vi "Main.vi"() -> ()   [LabVIEW 2017]
uses:
  1. CTL/DAQ_AO.ctl
  1. CTL/Controller.ctl
  <vilib>/DAQmx/read.llb/DAQmx Read (Analog 1D DBL 1Chan NSamp).vi
  <vilib>/Analysis/_algsub.llb/Real Vector Norm.vi
  <vilib>/DAQmx/write.llb/DAQmx Write (Digital Bool 1Line 1Point).vi
  <vilib>/DAQmx/write.llb/DAQmx Write (Analog 1D DBL 1Chan NSamp).vi
  <vilib>/DAQmx/write.llb/DAQmx Write (Analog 2D DBL NChan NSamp).vi
  <vilib>/Analysis/2dsp.llb/Decimate (single shot, DBL).vi
  <vilib>/DAQmx/create/channels.llb/DAQmx Create Channel (AO-Voltage-Basic).vi
  <vilib>/DAQmx/create/channels.llb/DAQmx Create Channel (AI-Voltage-Basic).vi
  <vilib>/DAQmx/configure/timing.llb/DAQmx Timing (Sample Clock).vi
  <vilib>/DAQmx/create/channels.llb/DAQmx Create Channel (DO-Digital Output).vi
  <vilib>/DAQmx/configure/trigger.llb/DAQmx Start Trigger (Analog Edge).vi
  <vilib>/DAQmx/miscellaneous.llb/DAQmx Fill In Error Info.vi
  <vilib>/Analysis/2dsp.llb/1D Cross Correlation (DBL).vi
  <vilib>/Analysis/NI_AALPro.lvlib
  <vilib>/Analysis/NI_AALBase.lvlib
panel:
  out "수신 신호 파형(PPM)":waveform(dbl)(graph)
  out "수신 신호 파형":waveform(dbl)(graph)
  out "최대값 3":dbl
  out "신호처리 파형(PPM)":waveform(dbl)(graph)
  out "최대값 2":dbl
  in  "Tab Control":T1(tab)
  in  "일시 정지 버튼":bool
  out "송신 신호생성 파형":waveform(dbl)[](graph)
  out "신호처리파형":waveform(dbl)(graph)
  out "최대값":dbl
  out "이전 최대값":dbl
  out "최대값 차이":dbl
  in  "정지 버튼":bool
  in  "수동시작 버튼":bool
  in  "자동시작 버튼":bool
  in  "Chip_rate_Threshold":u32(knob)=10 scale=0.0..20.0
  in  "Threshold":u32(knob)=10 scale=0.0..20.0
  in  "수신시간":dbl=0.5
  in  "Rc":dbl=5500.0 min=4000.0 step=100.0
  in  "Mask 데이터 참조 경로":string="C:\\Users\\FishingNetID\\Desktop\\TRX_CONTROLLER_SIMULATRO_1.4\\3. TDMS\\Coef8.tdms"
  in  "TX_Period":dbl=3.0
  in  "Mask 길이":enum16{"8 Order", "12 Order"}(ring)
  in  "주소":string="192.168.0.147"
  in  "원격 포트 또는 서비스 이름":u16=10000
  out "원소":T2
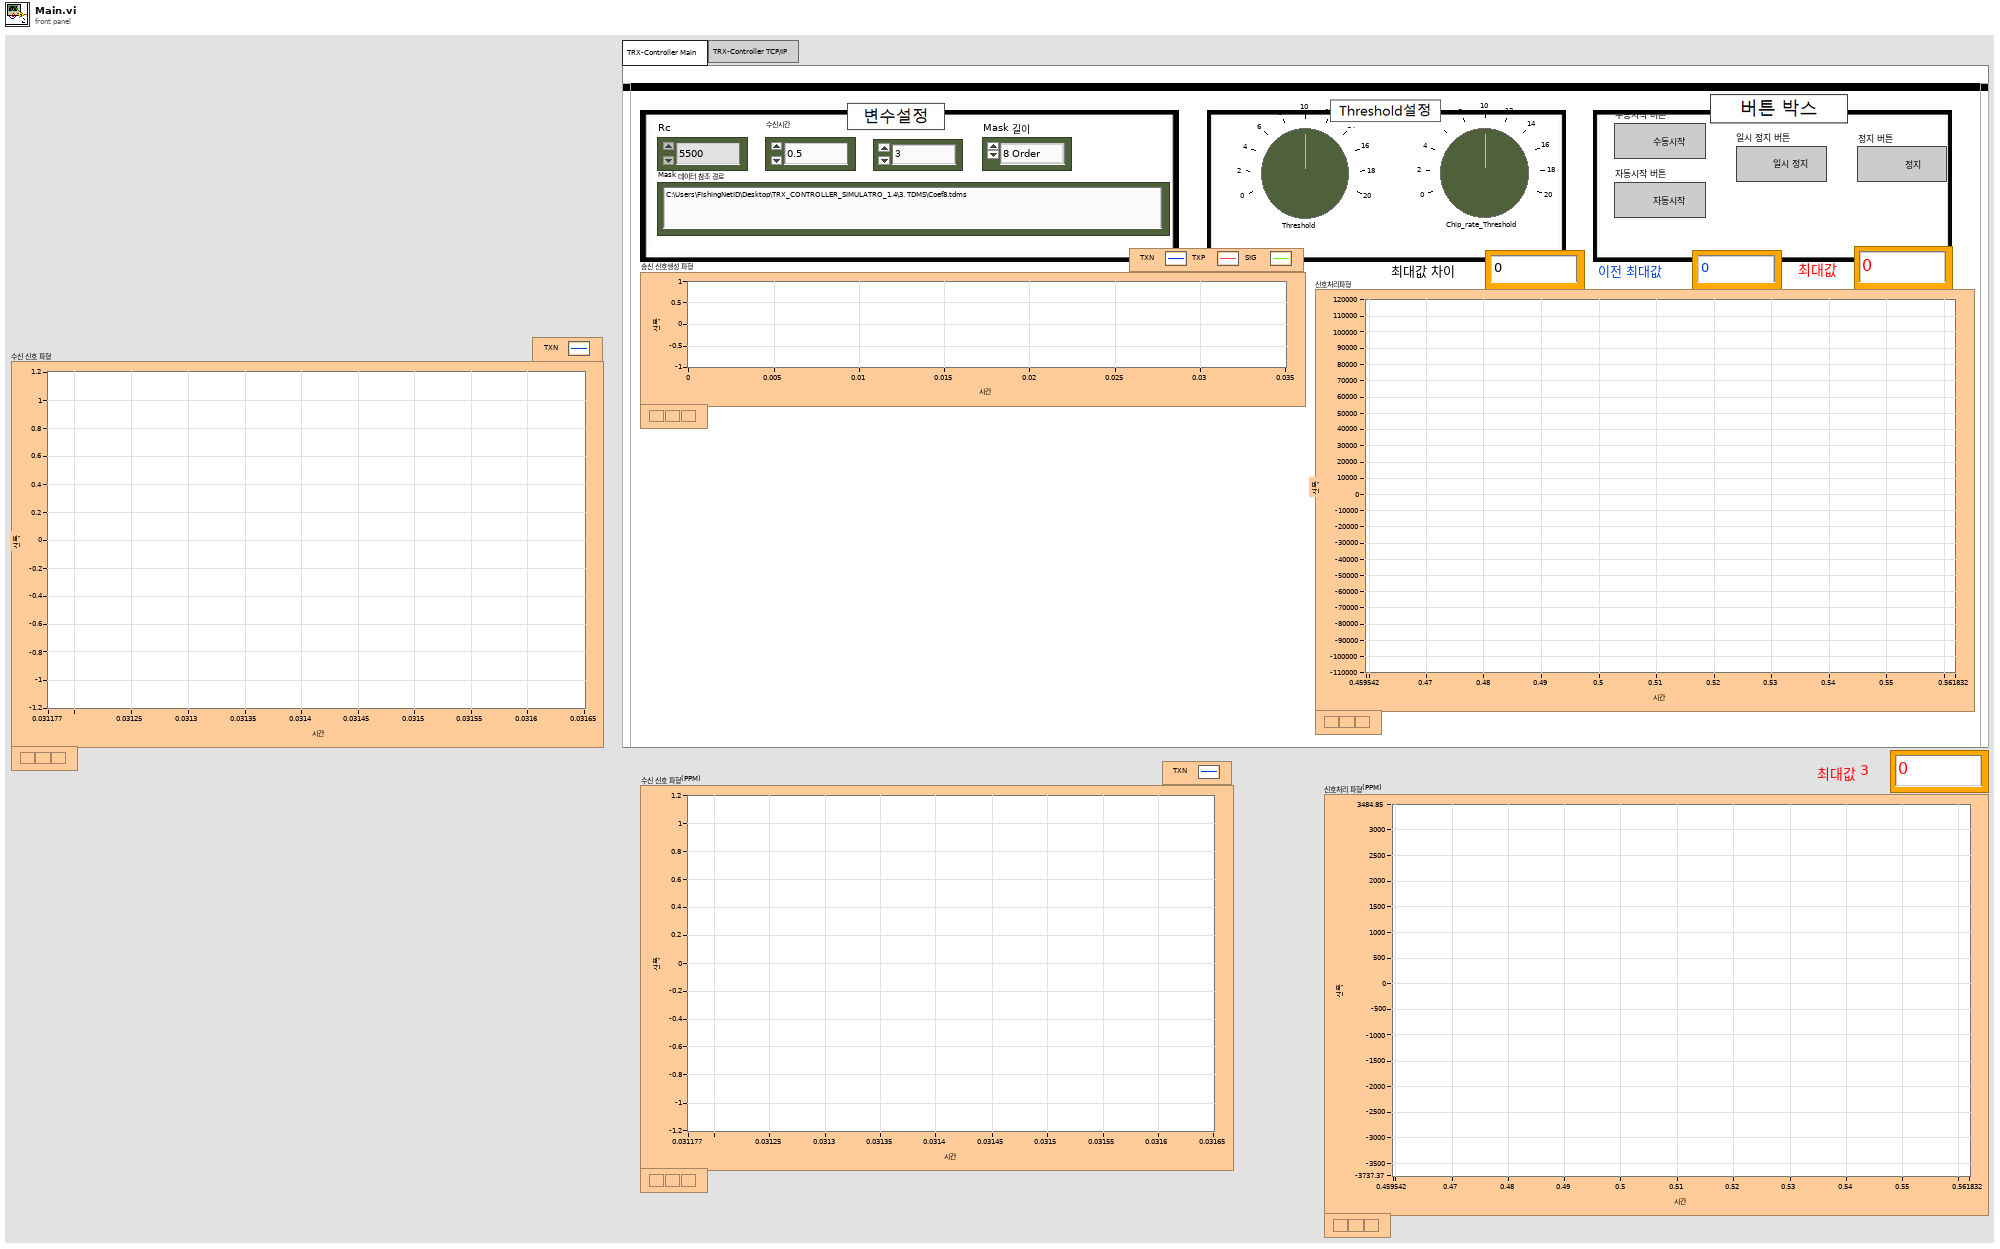
[diagram p1: front panel]
types:
  T1 = enum32{"TRX-Controller Main", "TRX-Controller TCP/IP"}
  T2 = typedef "DAQ_AO.ctl" = enum16{"통신 초기화", "통신 시작", "통신 정지"}
  T3 = cluster{"연결 ID":refnum<k5>, "TCP 에러":errorcluster}
  T4 = cluster{"송신신호 생성":waveform(dbl)[], "TXP 신호":dbl[], "TXN 신호":dbl[], "Fs":dbl, "AI 참조":refnum<k21>, "AO 참조":refnum<k21>, "수신시간":dbl, "Rc":dbl, "이전 최대값":dbl, "수신 신호처리 파형":waveform(dbl), "수신 파형":waveform(dbl), "최대값":dbl, "최대값 차이":dbl, "DO 참조":refnum<k21>, "TXEN 신호":bool[]}
  T5 = typedef "Controller.ctl" = enum16{"초기화", "수동시작", "신호처리", "정지", "값 변경", "일시정지", "자동시작"}
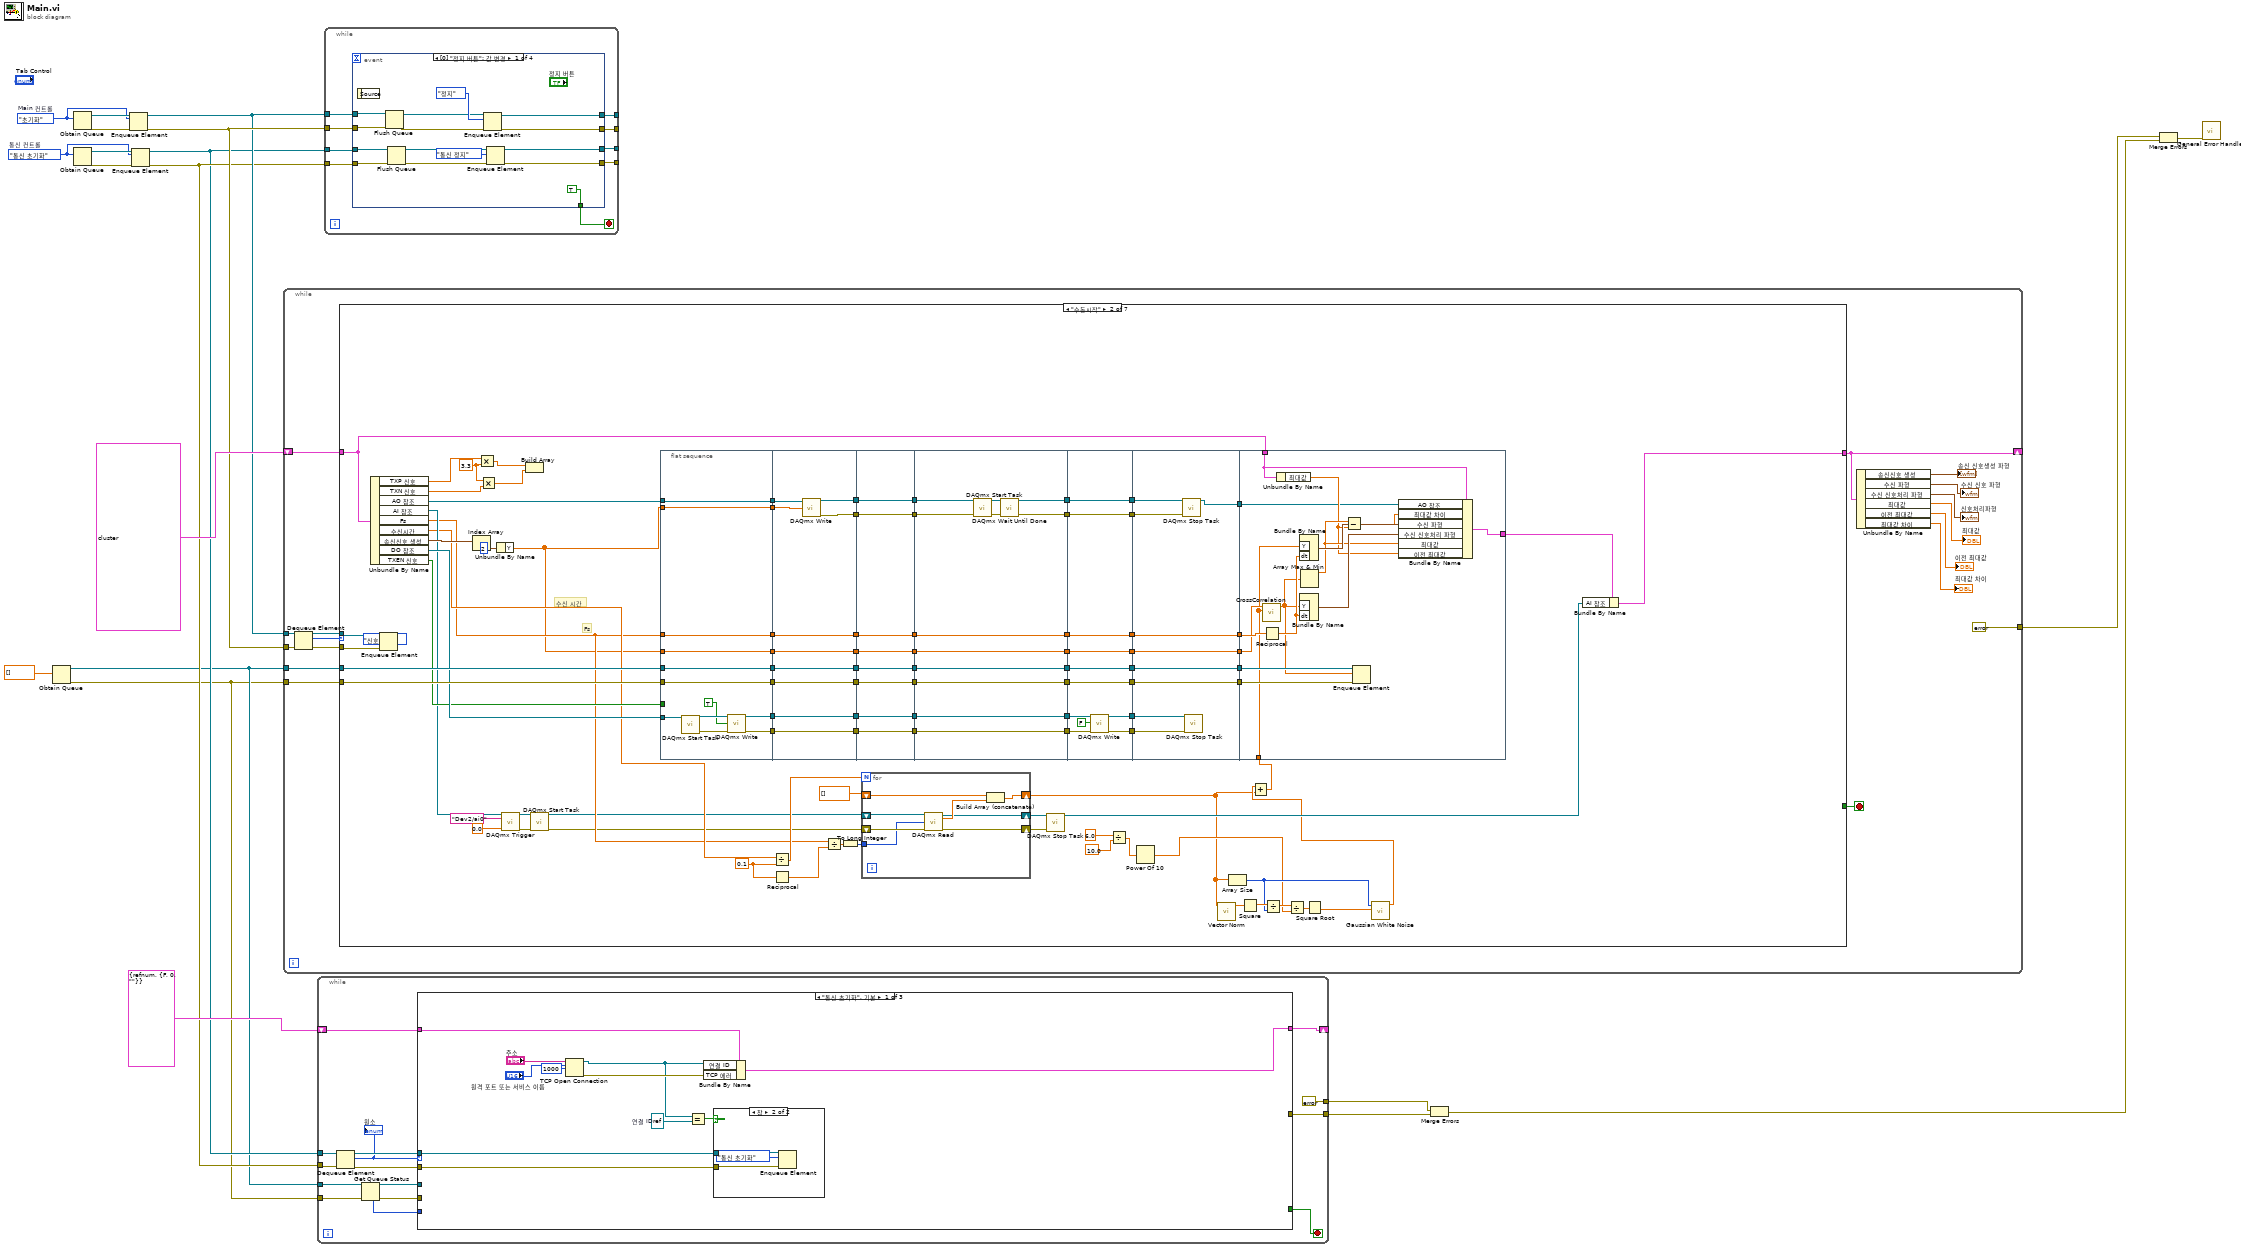
[diagram p0: block diagram]
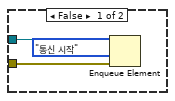
[diagram p2: hidden frame]
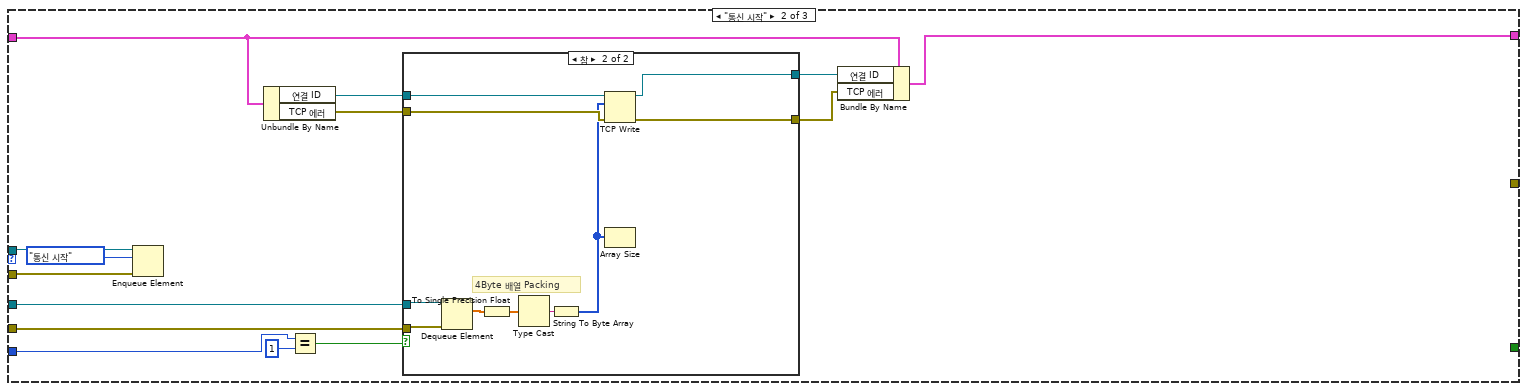
[diagram p3: hidden frame]
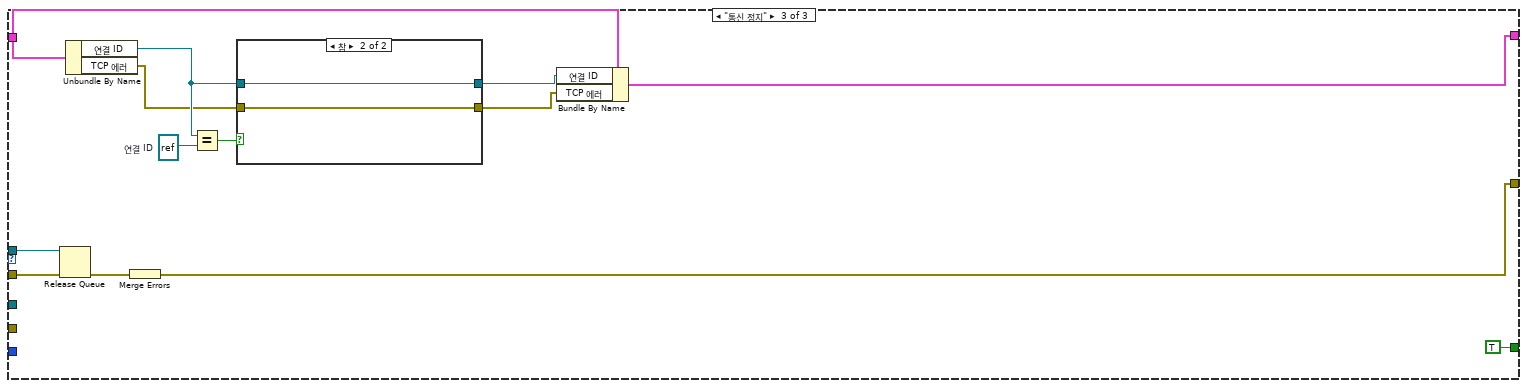
[diagram p5: hidden frame]
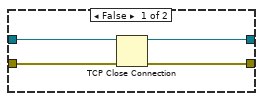
[diagram p6: hidden frame]
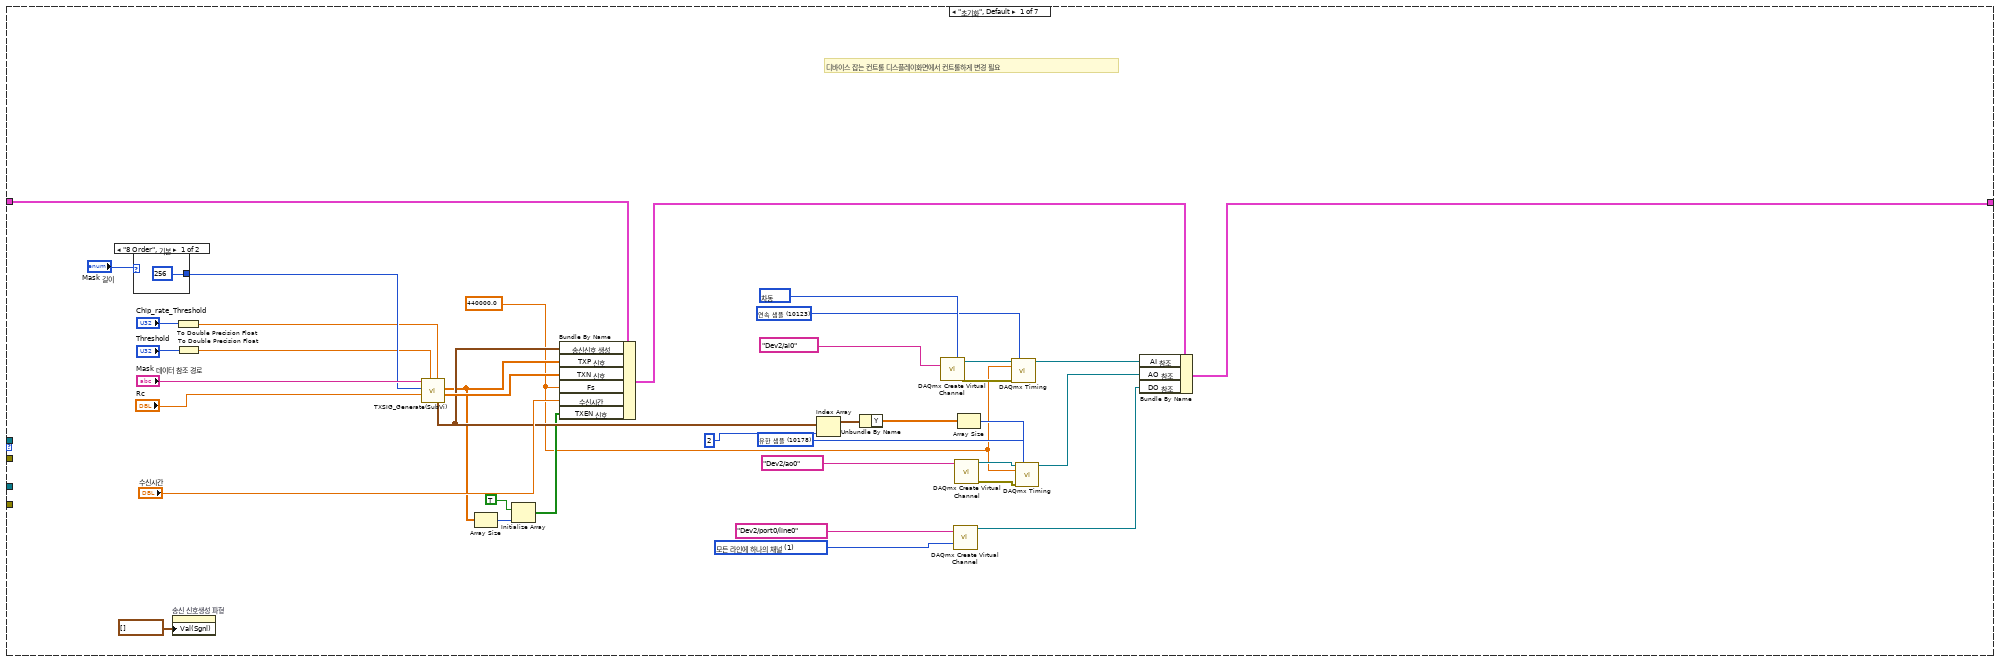
[diagram p7: hidden frame]
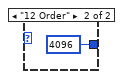
[diagram p8: hidden frame]
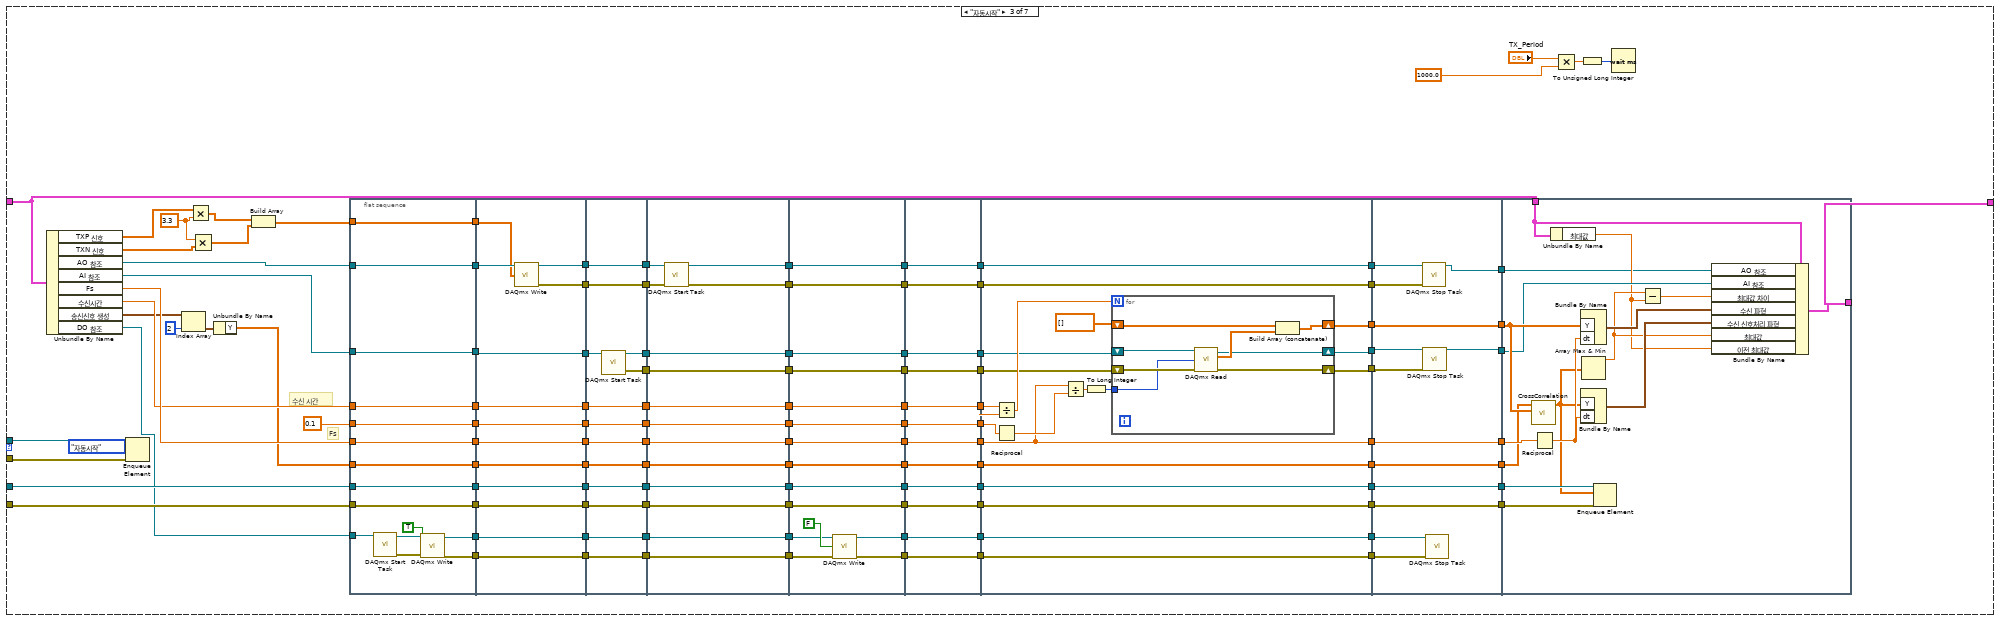
[diagram p9: hidden frame]
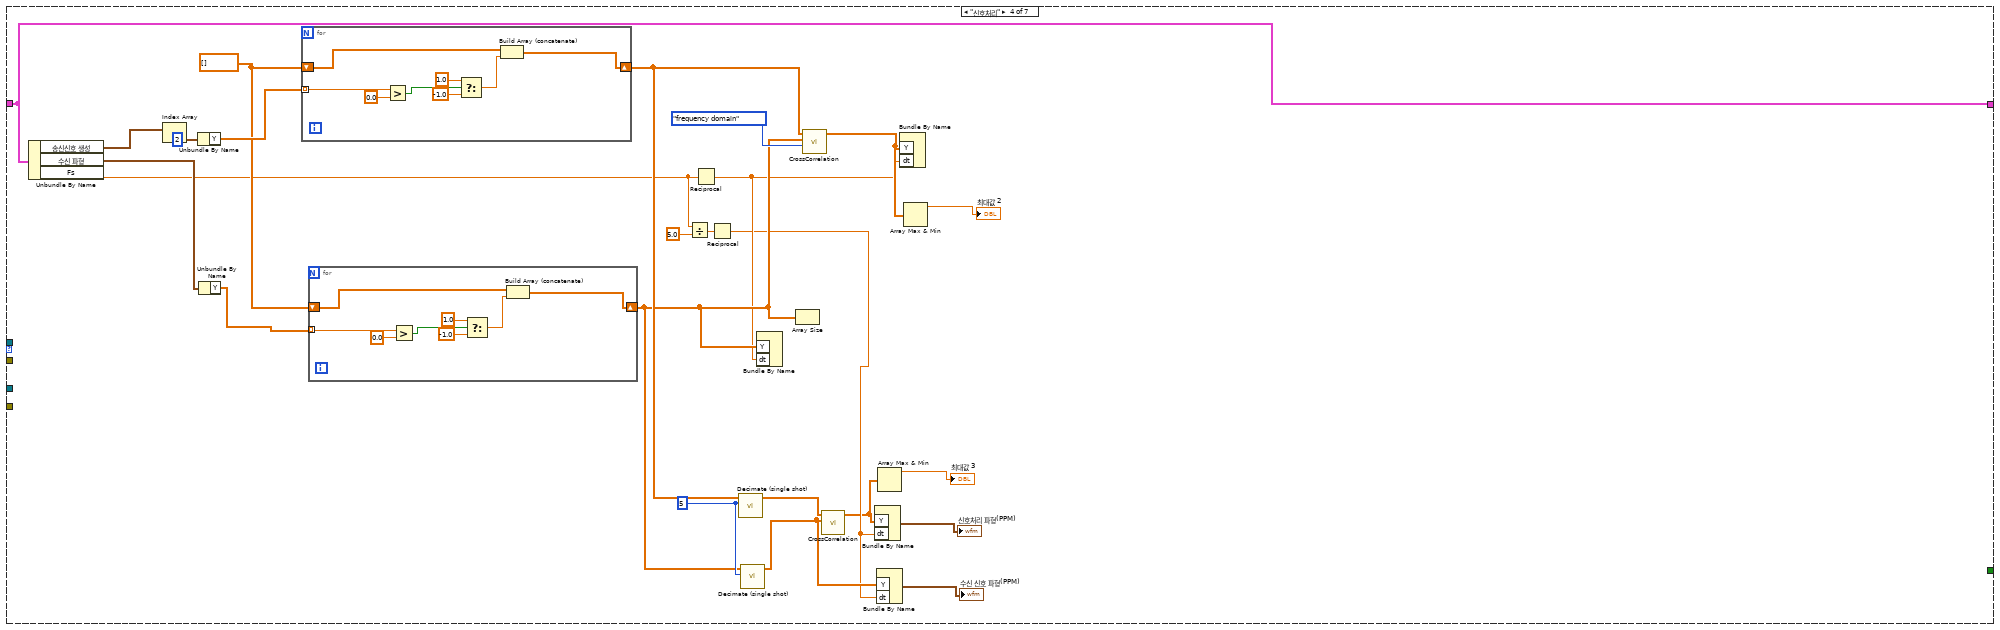
[diagram p10: hidden frame]
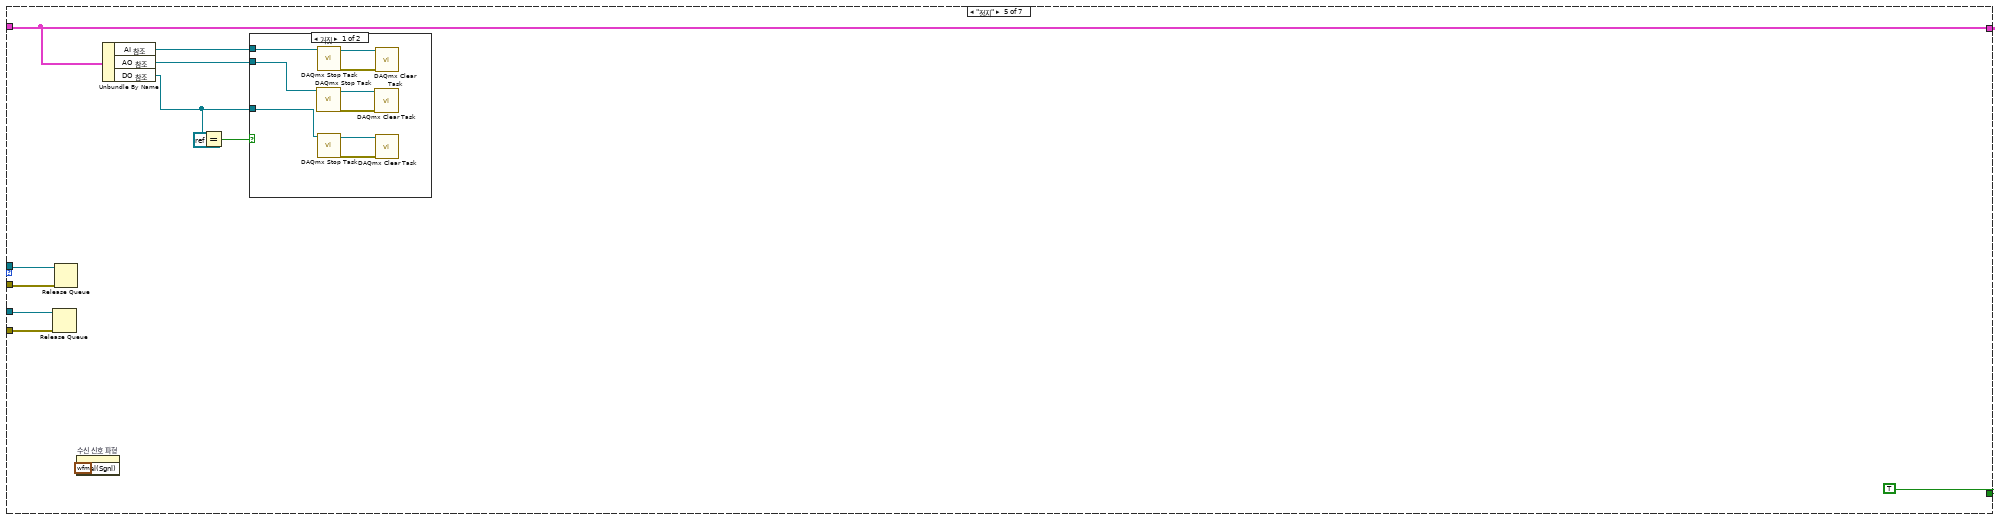
[diagram p11: hidden frame]
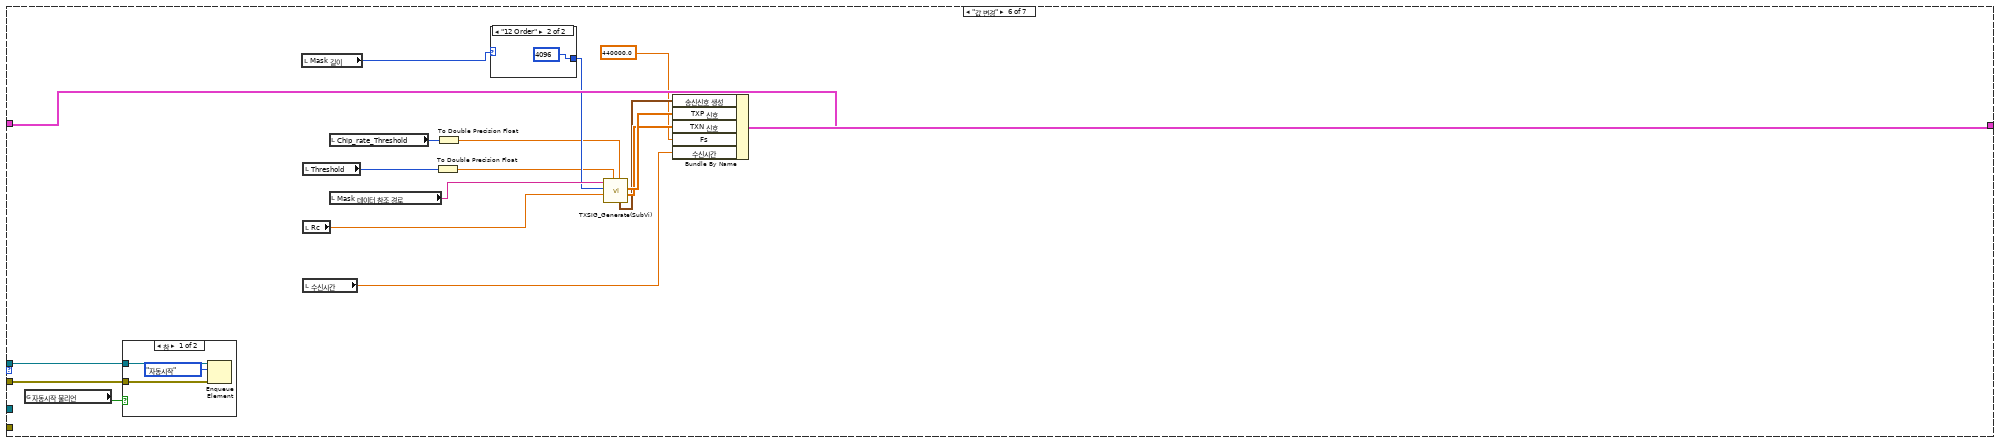
[diagram p13: hidden frame]
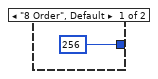
[diagram p14: hidden frame]
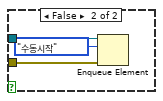
[diagram p15: hidden frame]
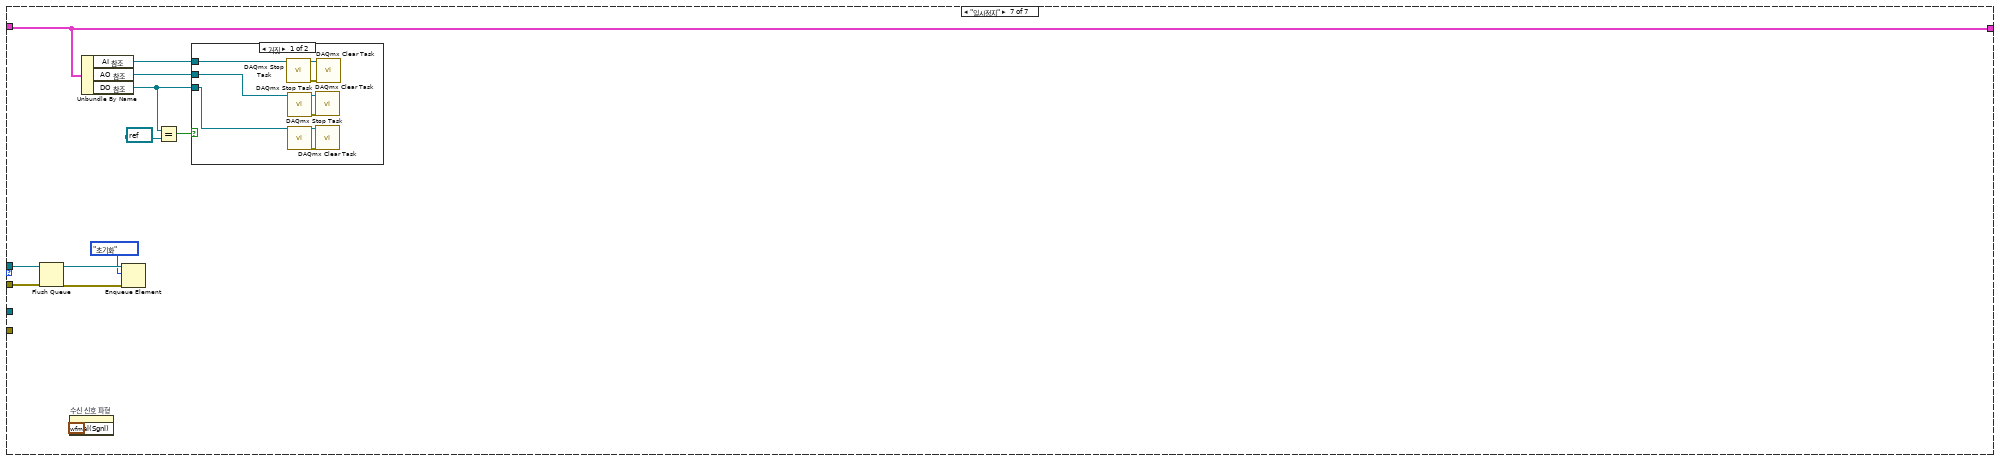
[diagram p16: hidden frame]
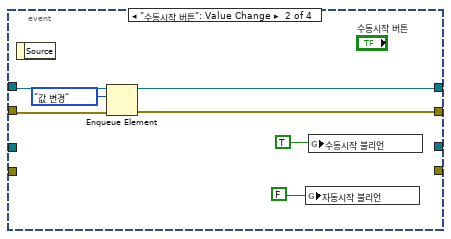
[diagram p18: hidden frame]
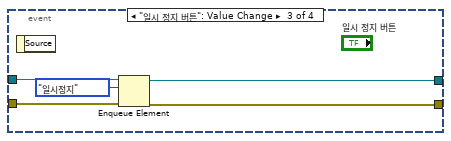
[diagram p19: hidden frame]
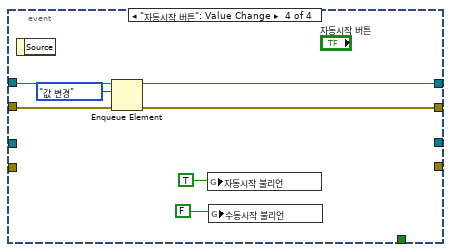
[diagram p20: hidden frame]
diagram:
  w8 = DAQ_AO."통신 초기화"  # 통신 컨트롤
  w15 = Controller."초기화"  # Main 컨트롤
  n1 = Obtain Queue(element data type=dbl[] []) -> (queue out=w2:refnum<queue>, error out=w1:errorcluster)  [unwired: 4 in, 1 out]
  n2 = Obtain Queue(element data type=w8) -> (queue out=w12:refnum<queue>, error out=w11:errorcluster)  [unwired: 4 in, 1 out]
  n3 = Obtain Queue(element data type=w15) -> (queue out=w19:refnum<queue>, error out=w18:errorcluster)  [unwired: 4 in, 1 out]
  n4 = Enqueue Element(queue=w19, element=w15, error in (no error)=w18) -> (queue out=w16:refnum<queue>, error out=w17:errorcluster)  [unwired: 1 in, 1 out]
  n5 = Enqueue Element(queue=w12, element=w8, error in (no error)=w11) -> (queue out=w9:refnum<queue>, error out=w10:errorcluster)  [unwired: 1 in, 1 out]
  n6 = while {
    tunnel: w16 -> [w37]
    tunnel: w17 -> [w36]
    tunnel: [errorcluster {"status"=FALSE, "code"=0, "source"=""} ("에러 상수")] -> w3
    shift-right: [w30] -> _
    shift-left: T4 {"송신신호 생성"=[], "TXP 신호"=[], "TXN 신호"=[], "Fs"=0.0, "AI 참조"="", "AO 참조"="", "수신시간"=0.0, "Rc"=0.0, "이전 최대값"=0.0, "수신 신호처리 파형"={"t0"=timestamp(0 s since 1904-01-01), "dt"=1.0, "Y"=[]}, "수신 파형"={"t0"=timestamp(0 s since 1904-01-01), "dt"=1.0, "Y"=[]}, "최대값"=0.0, "최대값 차이"=0.0, "DO 참조"="", "TXEN 신호"=[]} -> [w31]
    tunnel: w2 -> [w23]
    tunnel: w1 -> [w22]
    stop <- w34 stop-if-true
    n7 = Dequeue Element(queue=w37, error in (no error)=w36) -> (queue out=w33:refnum<queue>, element=w21:T5, error out=w32:errorcluster)  [unwired: 1 in, 1 out]
    n8 = case shown="\"수동시작\"" w21 {
      tunnel: [_ _ _ _ TRUE _ _] -> w34
      tunnel: w31 -> [w72 w172 w366 w531 w564 w584 w606]
      tunnel: [w73 w93 w345 w531 w564 w588 w606] -> w30
      tunnel: w33 -> [_ w135 w344 _ w555 w586 w612]
      tunnel: w32 -> [_ w134 w343 _ w554 w585 w611]
      tunnel: w23 -> [_ w162 w341 _ w557 _ _]
      tunnel: w22 -> [_ w160 w340 _ w556 _ _]
      frame "초기화", Default {
        w45 = 1 items=["각 라인에 하나의 채널", "모든 라인에 하나의 채널"] ("line grouping")
        w38 = 440000.0 ("Fs")
        w70 = 10106 items=["기본"=-1, "RSE"=10083, "NRSE"=10078, "차동"=10106, "유사 차동"=12529] ("input terminal configuration")
        w64 = 10178 items=["유한 샘플"=10178, "연속 샘플"=10123, "하드웨어 타이밍에 의한 단일 포인트"=12522] ("sample mode")
        w67 = 10123 items=["유한 샘플"=10178, "연속 샘플"=10123, "하드웨어 타이밍에 의한 단일 포인트"=12522] ("sample mode")
        # "디바이스 잡는 컨트롤 디스플레이화면에서 컨트롤하게 변경 필요"
        n9 = case shown="\"8 Order\", 기본" "Mask 길이" {
          tunnel: [256 4096] -> w55
          frame "8 Order", Default {
          }
          frame "12 Order" {
          }
        }
        n10 = property on="송신 신호생성 파형" class="WFGraph (엄격한)"("Val(Sgnl)"=waveform(dbl)[] []) -> ()  [unwired: 2 in, 2 out]
        n11 = To Double Precision Float(number="Chip_rate_Threshold") -> (double precision float=w53:dbl)
        n12 = To Double Precision Float(number="Threshold") -> (double precision float=w51:dbl)
        n13 = call "TXSIG_Generate(SubVi).vi"("Chip_rate_Threshold"=w53, "ThresHold"=w51, "Rc"="Rc", "길이"=w55, "이름 또는 상대 경로"="Mask 데이터 참조 경로") -> ("TXN"=w59:dbl[], "TXP"=w43:dbl[], "TXSIG"=w47:waveform(dbl)[])  [unwired: 4 in]
        n14 = Array Size(array=w43) -> (size(s)=w42:i32)
        n15 = Initialize Array(TRUE, w42) -> (w40:bool[])
        n16 = Bundle By Name(cluster=w72, "송신신호 생성"=w47, "TXP 신호"=w43, "TXN 신호"=w59, "Fs"=w38, "수신시간"="수신시간", "TXEN 신호"=w40) -> (w71:T4)
        n17 = Index Array(array=w47, index=2 ("인덱스")) -> (element=w49:waveform(dbl))
        n18 = Unbundle By Name(w49) -> ("Y"=w48:dbl[])
        n19 = call-poly <vilib>:"DAQmx Create Virtual Channel.vi"("input terminal configuration"=w70, "physical channels"=tag "Dev2/ai0") -> ("task out"=w69:refnum<k21>, "error out"=w68:errorcluster)  [unwired: 12 in]
        n20 = call-poly <vilib>:"DAQmx Create Virtual Channel.vi"("lines"=tag "Dev2/port0/line0", "line grouping"=w45) -> ("task out"=w44:refnum<k21>)  [unwired: 12 in, 1 out]
        n21 = call-poly <vilib>:"DAQmx Create Virtual Channel.vi"("physical channels"=tag "Dev2/ao0") -> ("task out"=w65:refnum<k21>, "error out"=w62:errorcluster)  [unwired: 13 in]
        n22 = Array Size(array=w48) -> (size(s)=w61:i32)
        n23 = call-poly <vilib>:"DAQmx Timing.vi"("task/channels in"=w69, "sample mode"=w67, "rate"=w38, "error in"=w68) -> ("task out"=w66:refnum<k21>)  [unwired: 10 in, 1 out]
        n24 = call-poly <vilib>:"DAQmx Timing.vi"("task/channels in"=w65, "sample mode"=w64, "samples per channel"=w61, "rate"=w38, "error in"=w62) -> ("task out"=w63:refnum<k21>)  [unwired: 9 in, 1 out]
        n25 = Bundle By Name(cluster=w71, "AI 참조"=w66, "AO 참조"=w63, "DO 참조"=w44) -> (w73:T4)
      }
      frame "수동시작" {
        w105 = 0.1 ("y")
        w167 = 3.3
        # "Fs"
        # "수신 시간"
        n26 = Unbundle By Name(w172) -> ("TXP 신호"=w169:dbl[], "TXN 신호"=w168:dbl[], "AO 참조"=w173:refnum<k21>, "AI 참조"=w113:refnum<k21>, "Fs"=w104:dbl, "수신시간"=w106:dbl, "송신신호 생성"=w165:waveform(dbl)[], "DO 참조"=w158:refnum<k21>, "TXEN 신호"=w142:bool[])
        n27 = Enqueue Element(queue=w135, element=Controller."신호처리" ("원소"), error in (no error)=w134) -> ()  [unwired: 1 in, 3 out]
        n28 = Index Array(array=w165, index=2 ("인덱스")) -> (element=w171:waveform(dbl))
        n29 = Multiply(x=w169, y=w167) -> (x*y=w143:dbl[])
        n30 = Multiply(x=w167, y=w168) -> (x*y=w166:dbl[])
        n31 = Unbundle By Name(w171) -> ("Y"=w91:dbl[])
        n32 = call-poly <vilib>:"DAQmx Trigger.vi"("task/channels in"=w113, "source"="Dev2/ai0", "level"=0.0) -> ("task out"=w115:refnum<k21>, "error out"=w114:errorcluster)  [unwired: 11 in]
        n33 = Build Array(w143, w166) -> ()  [unwired: 1 out]
        n34 = call <vilib>:"DAQmx Start Task.vi"("task/channels in"=w115, "error in"=w114) -> ("task out"=w103:refnum<k21>, "error out"=w102:errorcluster)  [unwired: 12 in]
        n35 = flat-sequence {
          tunnel: w158 -> [w187]
          tunnel: w160 -> [w188]
          tunnel: w162 -> [w189]
          tunnel: w91 -> [w190]
          tunnel: w91 -> [w191]
          tunnel: w104 -> [w192]
          tunnel: w173 -> [w193]
          tunnel: [w193] -> w157
          tunnel: [w192] -> w156
          tunnel: [w191] -> w155
          tunnel: [w190] -> w154
          tunnel: [w189] -> w153
          tunnel: [w188] -> w152
          tunnel: [w184] -> w147
          tunnel: [w183] -> w146
          tunnel: w142 -> [_]
          tunnel: [w202] -> w118
          tunnel: [w201] -> w120
          tunnel: [w200] -> w122
          tunnel: [w198] -> w124
          tunnel: [w197] -> w126
          tunnel: [w196] -> w128
          tunnel: w157 -> [w203]
          tunnel: w156 -> [w200]
          tunnel: w155 -> [w199]
          tunnel: w154 -> [w198]
          tunnel: w153 -> [w197]
          tunnel: w152 -> [w196]
          tunnel: [w195] -> w130
          tunnel: w147 -> [w195]
          tunnel: w146 -> [w194]
          tunnel: [w194] -> w132
          tunnel: w132 -> [w211]
          tunnel: [w211] -> w131
          tunnel: w130 -> [w210]
          tunnel: [w210] -> w129
          tunnel: w128 -> [w209]
          tunnel: [w209] -> w127
          tunnel: w126 -> [w208]
          tunnel: [w208] -> w125
          tunnel: w124 -> [w207]
          tunnel: [w207] -> w123
          tunnel: w122 -> [w206]
          tunnel: [w206] -> w121
          tunnel: w120 -> [w205]
          tunnel: [w205] -> w119
          tunnel: w118 -> [w204]
          tunnel: [w204] -> w117
          tunnel: [w223] -> w141
          tunnel: [w222] -> w140
          tunnel: [w221] -> w139
          tunnel: [w220] -> w138
          tunnel: [w219] -> w137
          tunnel: [w218] -> w136
          tunnel: w131 -> [w218]
          tunnel: w129 -> [w219]
          tunnel: w127 -> [w220]
          tunnel: w125 -> [w221]
          tunnel: w123 -> [w222]
          tunnel: w121 -> [w223]
          tunnel: w119 -> [w217]
          tunnel: w117 -> [w216]
          tunnel: [w213] -> w98
          tunnel: [w212] -> w97
          tunnel: w141 -> [w234]
          tunnel: [w234] -> w151
          tunnel: w140 -> [w233]
          tunnel: [w233] -> w150
          tunnel: w139 -> [w232]
          tunnel: [w232] -> w149
          tunnel: w138 -> [w231]
          tunnel: [w231] -> w148
          tunnel: w137 -> [w230]
          tunnel: w136 -> [w229]
          tunnel: [w228] -> w145
          tunnel: [w227] -> w144
          tunnel: [w225] -> w99
          tunnel: w98 -> [w225]
          tunnel: w97 -> [w224]
          tunnel: [w224] -> w96
          tunnel: [w243] -> w164
          tunnel: [w242] -> w163
          tunnel: [w241] -> w161
          tunnel: [w240] -> w159
          tunnel: [w237] -> w116
          tunnel: w151 -> [w243]
          tunnel: w150 -> [w242]
          tunnel: w149 -> [w241]
          tunnel: w148 -> [w240]
          tunnel: w145 -> [w239]
          tunnel: w144 -> [w238]
          tunnel: w99 -> [w236]
          tunnel: w96 -> [w235]
          tunnel: w172 -> [w255]
          tunnel: w164 -> [w257]
          tunnel: w163 -> [w256]
          tunnel: [w252] -> w95
          tunnel: w161 -> [w248]
          tunnel: w159 -> [w247]
          tunnel: w116 -> [w245]
          tunnel: w79 -> [w244]
          frame #0 {
            n36 = call <vilib>:"DAQmx Start Task.vi"("task/channels in"=w187) -> ("task out"=w186:refnum<k21>, "error out"=w185:errorcluster)  [unwired: 13 in]
            n37 = call-poly <vilib>:"DAQmx Write.vi"("task/channels in"=w186, "data"=TRUE, "error in"=w185) -> ("task out"=w184:refnum<k21>, "error out"=w183:errorcluster)  [unwired: 10 in, 1 out]
          }
          frame #1 {
            n38 = call-poly <vilib>:"DAQmx Write.vi"("task/channels in"=w203, "data"=w199) -> ("task out"=w202:refnum<k21>, "error out"=w201:errorcluster)  [unwired: 11 in, 1 out]
          }
          frame #2 {
          }
          frame #3 {
            n39 = call <vilib>:"DAQmx Start Task.vi"("task/channels in"=w216, "error in"=w217) -> ("task out"=w215:refnum<k21>, "error out"=w214:errorcluster)  [unwired: 12 in]
            n40 = call <vilib>:"DAQmx Wait Until Done.vi"("task/channels in"=w215, "error in"=w214) -> ("task out"=w213:refnum<k21>, "error out"=w212:errorcluster)  [unwired: 12 in]
          }
          frame #4 {
            n41 = call-poly <vilib>:"DAQmx Write.vi"("task/channels in"=w230, "data"=FALSE, "error in"=w229) -> ("task out"=w228:refnum<k21>, "error out"=w227:errorcluster)  [unwired: 10 in, 1 out]
          }
          frame #5 {
            n42 = call <vilib>:"DAQmx Stop Task.vi"("task/channels in"=w236, "error in"=w235) -> ("task out"=w237:refnum<k21>)  [unwired: 12 in, 1 out]
            n43 = call <vilib>:"DAQmx Stop Task.vi"("task/channels in"=w239, "error in"=w238) -> ()  [unwired: 12 in, 2 out]
          }
          frame #6 {
            n44 = call-poly <vilib>:"CrossCorrelation.vi"("Y"=w244, "X"=w256) -> ("Rxy"=w246:dbl[])  [unwired: 8 in, 1 out]
            n45 = Reciprocal(x=w257) -> (1/x=w258:dbl)
            n46 = Unbundle By Name(w255) -> ("최대값"=w249:dbl)
            n47 = Bundle By Name("Y"=w244, "dt"=w258) -> (w254:waveform(dbl))  [unwired: 1 in]
            n48 = Bundle By Name("Y"=w246, "dt"=w258) -> (w253:waveform(dbl))  [unwired: 1 in]
            n49 = Array Max & Min(array=w246) -> (max value=w250:dbl)  [unwired: 3 out]
            n50 = Subtract(x=w250, y=w249) -> (x-y=w251:dbl)
            n51 = Enqueue Element(queue=w248, element=w246, error in (no error)=w247) -> ()  [unwired: 1 in, 3 out]
            n52 = Bundle By Name(cluster=w255, "AO 참조"=w245, "최대값 차이"=w251, "수신 파형"=w254, "수신 신호처리 파형"=w253, "최대값"=w250, "이전 최대값"=w249) -> (w252:T4)
          }
        }
        n53 = Divide(x=w106, y=w105) -> (x/y=w108:dbl)
        n54 = Reciprocal(x=w105) -> (1/x=w109:dbl)
        n55 = Divide(x=w104, y=w109) -> (x/y=w111:dbl)
        n56 = To Long Integer(number=w111) -> (32bit integer=w110:i32)
        n57 = for {
          N: w108 -> [_]
          shift-right: [w179] -> w80
          shift-left: dbl[] [] -> [w181]
          shift-right: [w175] -> w101
          shift-left: w103 -> [w178]
          shift-right: [w176] -> w100
          shift-left: w102 -> [w177]
          tunnel: w110 -> [w174]
          n58 = call-poly <vilib>:"DAQmx Read.vi"("task/channels in"=w178, "number of samples per channel"=w174, "error in"=w177) -> ("task out"=w175:refnum<k21>, "data"=w180:dbl[], "error out"=w176:errorcluster)  [unwired: 10 in]
          n59 = Build Array (concatenate)(w181, w180) -> (w179:dbl[])
        }
        n60 = call <vilib>:"DAQmx Stop Task.vi"("task/channels in"=w101, "error in"=w100) -> ("task out"=w94:refnum<k21>)  [unwired: 12 in, 1 out]
        n61 = Divide(x=6.0, y=10.0) -> (x/y=w83:dbl)
        n62 = Power Of 10(x=w83) -> (10^x=w82:dbl)
        n63 = call-poly <vilib>:"Vector Norm.vi"("Input Vector"=w80) -> ("norm"=w89:dbl)  [unwired: 9 in, 1 out]
        n64 = Array Size(array=w80) -> (size(s)=w85:i32)
        n65 = Square(x=w89) -> (x^2=w88:dbl)
        n66 = Divide(x=w88, y=w85) -> (x/y=w87:dbl)
        n67 = Divide(x=w87, y=w82) -> (x/y=w86:dbl)
        n68 = Square Root(x=w86) -> (sqrt(x)=w84:dbl)
        n69 = call <vilib>:"Gaussian White Noise.vi"("standard deviation"=w84, "samples"=w85) -> ("Gaussian noise pattern"=w81:dbl[])  [unwired: 8 in, 1 out]
        n70 = Add(x=w81, y=w80) -> (x+y=w79:dbl[])
        n71 = Bundle By Name(cluster=w95, "AI 참조"=w94) -> (w93:T4)
      }
      frame "자동시작" {
        w358 = 3.3
        # "Fs"
        # "수신 시간"
        n72 = Unbundle By Name(w366) -> ("TXP 신호"=w360:dbl[], "TXN 신호"=w359:dbl[], "AO 참조"=w373:refnum<k21>, "AI 참조"=w354:refnum<k21>, "Fs"=w372:dbl, "수신시간"=w369:dbl, "송신신호 생성"=w355:waveform(dbl)[], "DO 참조"=w319:refnum<k21>)
        n73 = Enqueue Element(queue=w344, element=Controller."자동시작" ("원소"), error in (no error)=w343) -> ()  [unwired: 1 in, 3 out]
        n74 = Index Array(array=w355, index=2 ("인덱스")) -> (element=w362:waveform(dbl))
        n75 = Multiply(x=w360, y=w358) -> (x*y=w357:dbl[])
        n76 = Multiply(x=w358, y=w359) -> (x*y=w356:dbl[])
        n77 = Unbundle By Name(w362) -> ("Y"=w349:dbl[])
        n78 = Build Array(w357, w356) -> (w333:dbl[][])
        n79 = flat-sequence {
          tunnel: w333 -> [w380]
          tunnel: w340 -> [w381]
          tunnel: w341 -> [w382]
          tunnel: w349 -> [w383]
          tunnel: 0.1 ("y") -> [w384]
          tunnel: w369 -> [w385]
          tunnel: w372 -> [w386]
          tunnel: w354 -> [w387]
          tunnel: w373 -> [w388]
          tunnel: [w388] -> w328
          tunnel: [w387] -> w327
          tunnel: [w386] -> w326
          tunnel: [w385] -> w325
          tunnel: [w384] -> w324
          tunnel: [w383] -> w323
          tunnel: [w382] -> w322
          tunnel: [w381] -> w321
          tunnel: [w380] -> w320
          tunnel: w319 -> [w379]
          tunnel: [w375] -> w318
          tunnel: [w374] -> w316
          tunnel: [w400] -> w296
          tunnel: [w399] -> w294
          tunnel: [w398] -> w292
          tunnel: [w397] -> w290
          tunnel: [w396] -> w288
          tunnel: [w395] -> w286
          tunnel: [w394] -> w284
          tunnel: [w393] -> w282
          tunnel: w328 -> [w401]
          tunnel: w327 -> [w389]
          tunnel: w326 -> [w398]
          tunnel: w325 -> [w397]
          tunnel: w324 -> [w396]
          tunnel: w323 -> [w395]
          tunnel: w322 -> [w394]
          tunnel: w321 -> [w393]
          tunnel: w320 -> [w392]
          tunnel: w318 -> [w391]
          tunnel: [w391] -> w280
          tunnel: w316 -> [w390]
          tunnel: [w390] -> w278
          tunnel: [w389] -> w276
          tunnel: w296 -> [w414]
          tunnel: [w414] -> w295
          tunnel: w294 -> [w413]
          tunnel: [w413] -> w293
          tunnel: w292 -> [w412]
          tunnel: [w412] -> w291
          tunnel: w290 -> [w411]
          tunnel: [w411] -> w289
          tunnel: w288 -> [w410]
          tunnel: [w410] -> w287
          tunnel: w286 -> [w409]
          tunnel: [w409] -> w285
          tunnel: w284 -> [w408]
          tunnel: [w408] -> w283
          tunnel: w282 -> [w407]
          tunnel: [w407] -> w281
          tunnel: w280 -> [w406]
          tunnel: [w406] -> w279
          tunnel: w278 -> [w405]
          tunnel: [w405] -> w277
          tunnel: w276 -> [w404]
          tunnel: [w403] -> w272
          tunnel: [w402] -> w271
          tunnel: w295 -> [w422]
          tunnel: w293 -> [w421]
          tunnel: w291 -> [w428]
          tunnel: [w428] -> w370
          tunnel: [w427] -> w365
          tunnel: w289 -> [w427]
          tunnel: w287 -> [w426]
          tunnel: [w426] -> w352
          tunnel: [w425] -> w346
          tunnel: w285 -> [w425]
          tunnel: [w424] -> w337
          tunnel: w283 -> [w424]
          tunnel: [w423] -> w334
          tunnel: w281 -> [w423]
          tunnel: w279 -> [w420]
          tunnel: [w420] -> w317
          tunnel: w277 -> [w419]
          tunnel: [w419] -> w315
          tunnel: [w418] -> w273
          tunnel: w272 -> [w418]
          tunnel: w271 -> [w417]
          tunnel: [w417] -> w270
          tunnel: [w416] -> w267
          tunnel: [w415] -> w263
          tunnel: w370 -> [w443]
          tunnel: [w443] -> w312
          tunnel: [w442] -> w310
          tunnel: w365 -> [w442]
          tunnel: [w441] -> w308
          tunnel: w352 -> [w441]
          tunnel: [w440] -> w306
          tunnel: w346 -> [w440]
          tunnel: [w439] -> w304
          tunnel: w337 -> [w439]
          tunnel: [w438] -> w302
          tunnel: w334 -> [w438]
          tunnel: w317 -> [w436]
          tunnel: w315 -> [w435]
          tunnel: [w434] -> w300
          tunnel: [w433] -> w298
          tunnel: [w432] -> w274
          tunnel: w273 -> [w432]
          tunnel: w270 -> [w431]
          tunnel: [w431] -> w269
          tunnel: w267 -> [w430]
          tunnel: [w430] -> w266
          tunnel: w263 -> [w429]
          tunnel: [w429] -> w262
          tunnel: w312 -> [w455]
          tunnel: [w455] -> w311
          tunnel: w310 -> [w454]
          tunnel: [w454] -> w309
          tunnel: w308 -> [w453]
          tunnel: [w453] -> w307
          tunnel: w306 -> [w452]
          tunnel: [w452] -> w305
          tunnel: w304 -> [w451]
          tunnel: [w451] -> w303
          tunnel: w302 -> [w450]
          tunnel: [w450] -> w301
          tunnel: w300 -> [w449]
          tunnel: [w449] -> w299
          tunnel: w298 -> [w448]
          tunnel: [w448] -> w297
          tunnel: [w447] -> w275
          tunnel: w274 -> [w447]
          tunnel: w269 -> [w446]
          tunnel: [w446] -> w268
          tunnel: w266 -> [w445]
          tunnel: [w445] -> w265
          tunnel: w262 -> [w444]
          tunnel: [w444] -> w261
          tunnel: [w472] -> w371
          tunnel: w311 -> [w465]
          tunnel: w309 -> [w474]
          tunnel: [w471] -> w364
          tunnel: [w470] -> w363
          tunnel: w307 -> [w469]
          tunnel: [w465] -> w351
          tunnel: [w464] -> w347
          tunnel: w305 -> [w464]
          tunnel: [w463] -> w338
          tunnel: w303 -> [w463]
          tunnel: [w462] -> w335
          tunnel: w301 -> [w462]
          tunnel: w299 -> [w461]
          tunnel: [w461] -> w314
          tunnel: w297 -> [w460]
          tunnel: [w460] -> w313
          tunnel: w275 -> [w459]
          tunnel: w268 -> [w458]
          tunnel: w265 -> [w457]
          tunnel: [w457] -> w264
          tunnel: w261 -> [w456]
          tunnel: [w456] -> w260
          tunnel: w371 -> [w495]
          tunnel: [w494] -> w368
          tunnel: [w496] -> w367
          tunnel: w364 -> [w493]
          tunnel: w363 -> [w496]
          tunnel: w351 -> [w492]
          tunnel: [w492] -> w350
          tunnel: [w491] -> w348
          tunnel: w347 -> [w491]
          tunnel: [w490] -> w339
          tunnel: w338 -> [w490]
          tunnel: [w489] -> w336
          tunnel: w335 -> [w489]
          tunnel: w314 -> [w488]
          tunnel: w313 -> [w487]
          tunnel: w264 -> [w486]
          tunnel: w260 -> [w485]
          tunnel: [w484] -> w259
          tunnel: w366 -> [w508]
          tunnel: w350 -> [w510]
          tunnel: w367 -> [w511]
          tunnel: w368 -> [w507]
          tunnel: w348 -> [w509]
          tunnel: [w504] -> w345
          tunnel: w339 -> [w500]
          tunnel: w336 -> [w499]
          tunnel: w259 -> [w497]
          frame #0 {
            n80 = call <vilib>:"DAQmx Start Task.vi"("task/channels in"=w379) -> ("task out"=w377:refnum<k21>, "error out"=w378:errorcluster)  [unwired: 13 in]
            n81 = call-poly <vilib>:"DAQmx Write.vi"("task/channels in"=w377, "data"=TRUE, "error in"=w378) -> ("task out"=w375:refnum<k21>, "error out"=w374:errorcluster)  [unwired: 10 in, 1 out]
          }
          frame #1 {
            n82 = call-poly <vilib>:"DAQmx Write.vi"("task/channels in"=w401, "data"=w392) -> ("task out"=w400:refnum<k21>, "error out"=w399:errorcluster)  [unwired: 11 in, 1 out]
          }
          frame #2 {
            n83 = call <vilib>:"DAQmx Start Task.vi"("task/channels in"=w404) -> ("task out"=w403:refnum<k21>, "error out"=w402:errorcluster)  [unwired: 13 in]
          }
          frame #3 {
            n84 = call <vilib>:"DAQmx Start Task.vi"("task/channels in"=w422, "error in"=w421) -> ("task out"=w416:refnum<k21>, "error out"=w415:errorcluster)  [unwired: 12 in]
          }
          frame #4 {
            n85 = call-poly <vilib>:"DAQmx Write.vi"("task/channels in"=w436, "data"=FALSE, "error in"=w435) -> ("task out"=w434:refnum<k21>, "error out"=w433:errorcluster)  [unwired: 10 in, 1 out]
          }
          frame #5 {
          }
          frame #6 {
            n86 = Divide(x=w474, y=w469) -> (x/y=w473:dbl)
            n87 = Reciprocal(x=w469) -> (1/x=w468:dbl)
            n88 = Divide(x=w465, y=w468) -> (x/y=w466:dbl)
            n89 = To Long Integer(number=w466) -> (32bit integer=w467:i32)
            n90 = for {
              N: w473 -> [_]
              shift-right: [w481] -> w470
              shift-left: dbl[] [] -> [w483]
              shift-right: [w477] -> w472
              shift-left: w459 -> [w480]
              shift-right: [w478] -> w471
              shift-left: w458 -> [w479]
              tunnel: w467 -> [w476]
              n91 = call-poly <vilib>:"DAQmx Read.vi"("task/channels in"=w480, "number of samples per channel"=w476, "error in"=w479) -> ("task out"=w477:refnum<k21>, "data"=w482:dbl[], "error out"=w478:errorcluster)  [unwired: 10 in]
              n92 = Build Array (concatenate)(w483, w482) -> (w481:dbl[])
            }
          }
          frame #7 {
            n93 = call <vilib>:"DAQmx Stop Task.vi"("task/channels in"=w486, "error in"=w485) -> ("task out"=w484:refnum<k21>)  [unwired: 12 in, 1 out]
            n94 = call <vilib>:"DAQmx Stop Task.vi"("task/channels in"=w495, "error in"=w493) -> ("task out"=w494:refnum<k21>)  [unwired: 12 in, 1 out]
            n95 = call <vilib>:"DAQmx Stop Task.vi"("task/channels in"=w488, "error in"=w487) -> ()  [unwired: 12 in, 2 out]
          }
          frame #8 {
            n96 = call-poly <vilib>:"CrossCorrelation.vi"("Y"=w511, "X"=w509) -> ("Rxy"=w498:dbl[])  [unwired: 8 in, 1 out]
            n97 = Reciprocal(x=w510) -> (1/x=w512:dbl)
            n98 = Unbundle By Name(w508) -> ("최대값"=w501:dbl)
            n99 = Bundle By Name("Y"=w511, "dt"=w512) -> (w506:waveform(dbl))  [unwired: 1 in]
            n100 = Bundle By Name("Y"=w498, "dt"=w512) -> (w505:waveform(dbl))  [unwired: 1 in]
            n101 = Array Max & Min(array=w498) -> (max value=w502:dbl)  [unwired: 3 out]
            n102 = Enqueue Element(queue=w500, element=w498, error in (no error)=w499) -> ()  [unwired: 1 in, 3 out]
            n103 = Subtract(x=w502, y=w501) -> (x-y=w503:dbl)
            n104 = Bundle By Name(cluster=w508, "AO 참조"=w497, "AI 참조"=w507, "최대값 차이"=w503, "수신 파형"=w506, "수신 신호처리 파형"=w505, "최대값"=w502, "이전 최대값"=w501) -> (w504:T4)
          }
        }
        n105 = Multiply(x="TX_Period", y=1000.0) -> (x*y=w331:dbl)
        n106 = To Unsigned Long Integer(number=w331) -> (unsigned 32bit integer=w329:u32)
        n107 = Wait (ms)(milliseconds to wait=w329) -> ()  [unwired: 1 out]
      }
      frame "신호처리" {
        w525 = 5 ("decimating factor")
        w532 = dbl[] []
        n108 = Unbundle By Name(w531) -> ("송신신호 생성"=w537:waveform(dbl)[], "수신 파형"=w534:waveform(dbl), "Fs"=w518:dbl)
        n109 = Index Array(array=w537, index=2 ("인덱스")) -> (element=w535:waveform(dbl))
        n110 = Unbundle By Name(w535) -> ("Y"=w533:dbl[])
        n111 = Unbundle By Name(w534) -> ("Y"=w527:dbl[])
        n112 = for {
          shift-right: [w546] -> w526
          shift-left: w532 -> [w553]
          tunnel: w533 -> [w552] mode=indexing
          n113 = Greater?(x=w552, y=0.0) -> (0:w550:bool)
          n114 = Select(t=1.0, s=w550, f=-1.0) -> (s? t:f=w547:dbl)
          n115 = Build Array (concatenate)(w553, w547) -> (w546:dbl[])
        }
        n116 = for {
          shift-right: [w538] -> w524
          shift-left: w532 -> [w545]
          tunnel: w527 -> [w544] mode=indexing
          n117 = Greater?(x=w544, y=0.0) -> (0:w542:bool)
          n118 = Select(t=1.0, s=w542, f=-1.0) -> (s? t:f=w539:dbl)
          n119 = Build Array (concatenate)(w545, w539) -> (w538:dbl[])
        }
        n120 = Divide(x=w518, y=5.0) -> (x/y=w516:dbl)
        n121 = Reciprocal(x=w518) -> (1/x=w519:dbl)
        n122 = Reciprocal(x=w516) -> (1/x=w515:dbl)
        n123 = call-poly <vilib>:"Decimate (single shot).vi"("decimating factor"=w525, "X"=w526) -> ("Decimated Array"=w523:dbl[])  [unwired: 8 in, 1 out]
        n124 = call-poly <vilib>:"Decimate (single shot).vi"("decimating factor"=w525, "X"=w524) -> ("Decimated Array"=w520:dbl[])  [unwired: 8 in, 1 out]
        n125 = Bundle By Name("Y"=w524, "dt"=w519) -> ()  [unwired: 1 in, 1 out]
        n126 = Array Size(array=w524) -> ()  [unwired: 1 out]
        n127 = call-poly <vilib>:"CrossCorrelation.vi"("algorithm"=enum32{"direct", "frequency domain"}."frequency domain", "Y"=w524, "X"=w526) -> ("Rxy"=w530:dbl[])  [unwired: 7 in, 1 out]
        n128 = call-poly <vilib>:"CrossCorrelation.vi"("Y"=w520, "X"=w523) -> ("Rxy"=w513:dbl[])  [unwired: 8 in, 1 out]
        n129 = Bundle By Name("Y"=w513, "dt"=w515) -> (→"신호처리 파형(PPM)":waveform(dbl))  [unwired: 1 in]
        n130 = Bundle By Name("Y"=w520, "dt"=w515) -> (→"수신 신호 파형(PPM)":waveform(dbl))  [unwired: 1 in]
        n131 = Array Max & Min(array=w513) -> (max value=→"최대값 3":dbl)  [unwired: 3 out]
        n132 = Bundle By Name("Y"=w530, "dt"=w519) -> ()  [unwired: 1 in, 1 out]
        n133 = Array Max & Min(array=w530) -> (max value=→"최대값 2":dbl)  [unwired: 3 out]
      }
      frame "정지" {
        n134 = Release Queue(queue=w557, error in (no error)=w556) -> ()  [unwired: 1 in, 3 out]
        n135 = Release Queue(queue=w555, error in (no error)=w554) -> ()  [unwired: 1 in, 3 out]
        n136 = property on="수신 신호 파형" class="WFGraph (엄격한)"("Val(Sgnl)"=waveform(dbl) {"t0"=timestamp(0 s since 1904-01-01), "dt"=1.0, "Y"=[]} ("Waveform")) -> ()  [unwired: 2 in, 2 out]
        n137 = Unbundle By Name(w564) -> ("AI 참조"=w563:refnum<k21>, "AO 참조"=w562:refnum<k21>, "DO 참조"=w558:refnum<k21>)
        n138 = Equal?(x=w558, y=refnum<k21> refnum) -> (x = y?=w560:bool)
        n139 = case shown="거짓" w560 {
          tunnel: w563 -> [w572 _]
          tunnel: w562 -> [w569 _]
          tunnel: w558 -> [w566 _]
          frame False {
            n140 = call <vilib>:"DAQmx Stop Task.vi"("task/channels in"=w569) -> ("task out"=w570:refnum<k21>, "error out"=w571:errorcluster)  [unwired: 13 in]
            n141 = call <vilib>:"DAQmx Stop Task.vi"("task/channels in"=w572) -> ("task out"=w574:refnum<k21>, "error out"=w573:errorcluster)  [unwired: 13 in]
            n142 = call <vilib>:"DAQmx Stop Task.vi"("task/channels in"=w566) -> ("task out"=w568:refnum<k21>, "error out"=w567:errorcluster)  [unwired: 13 in]
            n143 = call <vilib>:"DAQmx Clear Task.vi"("task in"=w570, "error in"=w571) -> ()  [unwired: 13 in, 1 out]
            n144 = call <vilib>:"DAQmx Clear Task.vi"("task in"=w574, "error in"=w573) -> ()  [unwired: 13 in, 1 out]
            n145 = call <vilib>:"DAQmx Clear Task.vi"("task in"=w568, "error in"=w567) -> ()  [unwired: 13 in, 1 out]
          }
          frame True {
          }
        }
      }
      frame "값 변경" {
        n146 = global read "시작 글로벌.vi" "자동시작 불리언"() -> (w587:bool)
        n147 = case shown="참" w587 {
          tunnel: w586 -> [w597 w600]
          tunnel: w585 -> [w596 w599]
          frame True {
            n148 = Enqueue Element(queue=w597, element=Controller."자동시작" ("원소"), error in (no error)=w596) -> ()  [unwired: 1 in, 3 out]
          }
          frame False {
            n149 = Enqueue Element(queue=w600, element=Controller."수동시작" ("원소"), error in (no error)=w599) -> ()  [unwired: 1 in, 3 out]
          }
        }
        n150 = local read "Mask 길이"() -> (w583:enum16{"8 Order", "12 Order"})
        n151 = local read "Threshold"() -> (w579:u32)
        n152 = local read "Rc"() -> (w576:dbl)
        n153 = local read "수신시간"() -> (w590:dbl)
        n154 = local read "Chip_rate_Threshold"() -> (w581:u32)
        n155 = local read "Mask 데이터 참조 경로"() -> (w589:string)
        n156 = To Double Precision Float(number=w579) -> (double precision float=w578:dbl)
        n157 = To Double Precision Float(number=w581) -> (double precision float=w580:dbl)
        n158 = case shown="\"12 Order\"" w583 {
          tunnel: [256 4096] -> w582
          frame "8 Order", Default {
          }
          frame "12 Order" {
          }
        }
        n159 = call "TXSIG_Generate(SubVi).vi"("Chip_rate_Threshold"=w580, "ThresHold"=w578, "Rc"=w576, "길이"=w582, "이름 또는 상대 경로"=w589) -> ("TXN"=w591:dbl[], "TXP"=w592:dbl[], "TXSIG"=w577:waveform(dbl)[])  [unwired: 4 in]
        n160 = Bundle By Name(cluster=w584, "송신신호 생성"=w577, "TXP 신호"=w592, "TXN 신호"=w591, "Fs"=440000.0, "수신시간"=w590) -> (w588:T4)
      }
      frame "일시정지" {
        n161 = Flush Queue(queue=w612, error in (no error)=w611) -> (queue out=w605:refnum<queue>, error out=w604:errorcluster)  [unwired: 1 out]
        n162 = property on="수신 신호 파형" class="WFGraph (엄격한)"("Val(Sgnl)"=waveform(dbl) {"t0"=timestamp(0 s since 1904-01-01), "dt"=1.0, "Y"=[]} ("Waveform")) -> ()  [unwired: 2 in, 2 out]
        n163 = Unbundle By Name(w606) -> ("AI 참조"=w607:refnum<k21>, "AO 참조"=w608:refnum<k21>, "DO 참조"=w601:refnum<k21>)
        n164 = Enqueue Element(queue=w605, element=Controller."초기화" ("원소"), error in (no error)=w604) -> ()  [unwired: 1 in, 3 out]
        n165 = Equal?(x=w601, y=refnum<k21> refnum) -> (x = y?=w609:bool)
        n166 = case shown="거짓" w609 {
          tunnel: w608 -> [w620 _]
          tunnel: w607 -> [w621 _]
          tunnel: w601 -> [w614 _]
          frame False {
            n167 = call <vilib>:"DAQmx Stop Task.vi"("task/channels in"=w621) -> ("task out"=w619:refnum<k21>, "error out"=w618:errorcluster)  [unwired: 13 in]
            n168 = call <vilib>:"DAQmx Stop Task.vi"("task/channels in"=w620) -> ("task out"=w617:refnum<k21>, "error out"=w616:errorcluster)  [unwired: 13 in]
            n169 = call <vilib>:"DAQmx Stop Task.vi"("task/channels in"=w614) -> ("task out"=w613:refnum<k21>, "error out"=w615:errorcluster)  [unwired: 13 in]
            n170 = call <vilib>:"DAQmx Clear Task.vi"("task in"=w617, "error in"=w616) -> ()  [unwired: 13 in, 1 out]
            n171 = call <vilib>:"DAQmx Clear Task.vi"("task in"=w613, "error in"=w615) -> ()  [unwired: 13 in, 1 out]
            n172 = call <vilib>:"DAQmx Clear Task.vi"("task in"=w619, "error in"=w618) -> ()  [unwired: 13 in, 1 out]
          }
          frame True {
          }
        }
      }
    }
    n173 = Unbundle By Name(w30) -> ("송신신호 생성"=→"송신 신호생성 파형":waveform(dbl)[], "수신 파형"=→"수신 신호 파형":waveform(dbl), "수신 신호처리 파형"=→"신호처리파형":waveform(dbl), "최대값"=→"최대값":dbl, "이전 최대값"=→"이전 최대값":dbl, "최대값 차이"=→"최대값 차이":dbl)
  }
  n174 = while {
    tunnel: w9 -> [w636]
    tunnel: w10 -> [w635]
    shift-right: [w630] -> _
    shift-left: T3 {"연결 ID"=refnum, "TCP 에러"={"status"=FALSE, "code"=0, "source"=""}} -> [w631]
    tunnel: w2 -> [w625]
    tunnel: w1 -> [w624]
    tunnel: [errorcluster {"status"=FALSE, "code"=0, "source"=""} ("에러 상수")] -> w6
    tunnel: [w622] -> w4
    stop <- w632 stop-if-true
    n175 = Dequeue Element(queue=w636, error in (no error)=w635) -> (queue out=w634:refnum<queue>, element=w628:T2, error out=w633:errorcluster)  [unwired: 1 in, 1 out]
    "원소" <- w628
    n176 = Get Queue Status(queue=w625, error in (no error)=w624) -> (queue out=w627:refnum<queue>, error out=w626:errorcluster, # elements in queue=w623:i32)  [unwired: 1 in, 5 out]
    n177 = case shown="\"통신 초기화\", 기본" w628 {
      tunnel: w634 -> [w638 w665 w683]
      tunnel: w633 -> [w637 w664 w682]
      tunnel: [_ _ TRUE] -> w632
      tunnel: w631 -> [w647 w667 w687]
      tunnel: [w646 w666 w684] -> w630
      tunnel: w627 -> [_ w656 _]
      tunnel: w626 -> [_ w655 _]
      tunnel: w623 -> [_ w654 _]
      tunnel: [_ _ w680] -> w622
      frame "통신 초기화", Default {
        w640 = refnum<k5> refnum  # 연결 ID
        n178 = TCP Open Connection(address="주소", remote port or service name="원격 포트 또는 서비스 이름", timeout ms (60000)=1000 ("타임아웃 ms (60000)")) -> (connection ID=w641:refnum<k5>, error out=w643:errorcluster)  [unwired: 2 in]
        n179 = Equal?(x=w641, y=w640) -> (x = y?=w639:bool)
        n180 = Bundle By Name(cluster=w647, "연결 ID"=w641, "TCP 에러"=w643) -> (w646:T3)
        n181 = case shown="참" w639 {
          tunnel: w638 -> [w650 w653]
          tunnel: w637 -> [w649 w652]
          frame False {
            n182 = Enqueue Element(queue=w650, element=DAQ_AO."통신 시작" ("원소"), error in (no error)=w649) -> ()  [unwired: 1 in, 3 out]
          }
          frame True {
            n183 = Enqueue Element(queue=w653, element=DAQ_AO."통신 초기화" ("원소"), error in (no error)=w652) -> ()  [unwired: 1 in, 3 out]
          }
        }
      }
      frame "통신 시작" {
        n184 = Enqueue Element(queue=w665, element=DAQ_AO."통신 시작" ("원소"), error in (no error)=w664) -> ()  [unwired: 1 in, 3 out]
        n185 = Unbundle By Name(w667) -> ("연결 ID"=w660:refnum<k5>, "TCP 에러"=w659:errorcluster)
        n186 = Equal?(x=w654, y=1) -> (x = y?=w662:bool)
        n187 = case shown="참" w662 {
          tunnel: w656 -> [_ w679]
          tunnel: w655 -> [_ w678]
          tunnel: w660 -> [w669 w676]
          tunnel: w659 -> [w668 w675]
          tunnel: [w669 w674] -> w658
          tunnel: [w668 w673] -> w657
          frame False {
          }
          frame True {
            # "4Byte 배열 Packing"
            n188 = Dequeue Element(queue=w679, error in (no error)=w678) -> (element=w671:dbl[])  [unwired: 1 in, 3 out]
            n189 = To Single Precision Float(number=w671) -> (single precision float=w670:sgl[])
            n190 = Type Cast(x=w670) -> (*(type *) &x=w677:string)  [unwired: 1 in]
            n191 = String To Byte Array(string=w677) -> (unsigned byte array=w672:u8[])
            n192 = TCP Write(connection ID=w676, data in=w672, error in (no error)=w675) -> (connection ID out=w674:refnum<k5>, error out=w673:errorcluster)  [unwired: 1 in, 1 out]
            n193 = Array Size(array=w672) -> ()  [unwired: 1 out]
          }
        }
        n194 = Bundle By Name(cluster=w667, "연결 ID"=w658, "TCP 에러"=w657) -> (w666:T3)
      }
      frame "통신 정지" {
        w691 = refnum<k5> refnum  # 연결 ID
        n195 = Release Queue(queue=w683, error in (no error)=w682) -> (error out=w681:errorcluster)  [unwired: 1 in, 2 out]
        n196 = Unbundle By Name(w687) -> ("연결 ID"=w689:refnum<k5>, "TCP 에러"=w688:errorcluster)
        n197 = Merge Errors(w681) -> (w680:errorcluster)
        n198 = Equal?(x=w689, y=w691) -> (x = y?=w690:bool)
        n199 = case shown="참" w690 {
          tunnel: w689 -> [w696 w698]
          tunnel: w688 -> [w695 w697]
          tunnel: [w694 w698] -> w686
          tunnel: [w693 w697] -> w685
          frame False {
            n200 = TCP Close Connection(connection ID=w696, error in (no error)=w695) -> (connection ID out=w694:refnum<k5>, error out=w693:errorcluster)  [unwired: 1 in]
          }
          frame True {
          }
        }
        n201 = Bundle By Name(cluster=w687, "연결 ID"=w686, "TCP 에러"=w685) -> (w684:T3)
      }
    }
  }
  n202 = while {
    tunnel: w17 -> [w707]
    tunnel: w16 -> [w706]
    tunnel: [w704] -> _
    tunnel: [w703] -> _
    tunnel: w9 -> [w702]
    tunnel: w10 -> [w701]
    tunnel: [w700] -> _
    tunnel: [w699] -> _
    stop <- w705 stop-if-true
    n203 = event shown="[0] \"정지 버튼\": 값 변경" {
      selector: _ -> [_ _ _ _]
      dyn-events: _ -> [_ _ _ _]
      timeout: _ -> [_ _ _ _]
      tunnel: w707 -> [w717 w728 w733 w740]
      tunnel: w706 -> [w718 w729 w734 w741]
      tunnel: [TRUE _ _ _] -> w705
      tunnel: [w720 w723 w730 w735] -> w704
      tunnel: [w719 w724 w731 w736] -> w703
      tunnel: w702 -> [w711 _ _ _]
      tunnel: w701 -> [w710 _ _ _]
      tunnel: [w709 _ _ _] -> w700
      tunnel: [w708 _ _ _] -> w699
      event "정지 버튼": Value Change {
        n204 = event-data() -> ()  [unwired: 1 in, 1 out]
        n205 = Flush Queue(queue=w718, error in (no error)=w717) -> (queue out=w716:refnum<queue>, error out=w715:errorcluster)  [unwired: 1 out]
        n206 = Flush Queue(queue=w711, error in (no error)=w710) -> (queue out=w714:refnum<queue>, error out=w713:errorcluster)  [unwired: 1 out]
        n207 = Enqueue Element(queue=w716, element=Controller."정지" ("원소"), error in (no error)=w715) -> (queue out=w719:refnum<queue>, error out=w720:errorcluster)  [unwired: 1 in, 1 out]
        n208 = Enqueue Element(queue=w714, element=DAQ_AO."통신 정지" ("원소"), error in (no error)=w713) -> (queue out=w709:refnum<queue>, error out=w708:errorcluster)  [unwired: 1 in, 1 out]
      }
      event "수동시작 버튼": Value Change {
        n209 = event-data() -> ()  [unwired: 1 in, 1 out]
        n210 = Enqueue Element(queue=w729, element=Controller."값 변경" ("원소"), error in (no error)=w728) -> (queue out=w724:refnum<queue>, error out=w723:errorcluster)  [unwired: 1 in, 1 out]
        n211 = global write "시작 글로벌.vi" "자동시작 불리언"(FALSE) -> ()
        n212 = global write "시작 글로벌.vi" "수동시작 불리언"(TRUE) -> ()
      }
      event "일시 정지 버튼": Value Change {
        n213 = event-data() -> ()  [unwired: 1 in, 1 out]
        n214 = Enqueue Element(queue=w734, element=Controller."일시정지" ("원소"), error in (no error)=w733) -> (queue out=w731:refnum<queue>, error out=w730:errorcluster)  [unwired: 1 in, 1 out]
      }
      event "자동시작 버튼": Value Change {
        n215 = event-data() -> ()  [unwired: 1 in, 1 out]
        n216 = Enqueue Element(queue=w741, element=Controller."값 변경" ("원소"), error in (no error)=w740) -> (queue out=w736:refnum<queue>, error out=w735:errorcluster)  [unwired: 1 in, 1 out]
        n217 = global write "시작 글로벌.vi" "자동시작 불리언"(TRUE) -> ()
        n218 = global write "시작 글로벌.vi" "수동시작 불리언"(FALSE) -> ()
      }
    }
  }
  n219 = Merge Errors(w6, w4) -> (w5:errorcluster)
  n220 = Merge Errors(w3, w5) -> (w7:errorcluster)
  n221 = call <vilib>:"General Error Handler.vi"("error in (no error)"=w7) -> ()  [unwired: 10 in, 5 out]
